vi "Teleop.vi"(10 "Match Info":T1={"Autonomous Elapsed Seconds"=0.0, "TeleOp Elapsed Seconds"=0.0, "Disabled Elapsed Seconds"=0.0, "Visited Autonomous"=FALSE, "Visited TeleOp"=FALSE, "Visited Disabled"=FALSE, "Autonomous Settings"={"Autonomous Style"=enum."Independent", "VI Refnum"=refnum}}, 11 "Call Context":T2) -> ()   [LabVIEW 2019]
doc: "This VI is called for each TeleOp packet received from the DS where the robot is not disabled. It is often used to read from the joysticks and update I/O or to update setpoints for timed control loops. It should complete and return within 20 milliseconds or it may miss DS packets."
uses:
  <vilib>/Rock Robotics/WPI/DriverStation/WPI_DriverStationDerivedRobotMode.ctl
  <vilib>/Rock Robotics/WPI/DriverStation/WPI_DriverStationMatch Info.ctl
  <vilib>/Rock Robotics/WPI/Utilities/WPI_GetSetVariantRefNum.vi
  Robot Global Data.vi
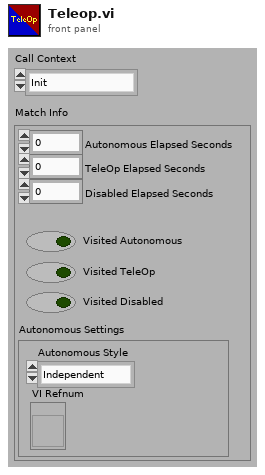
[diagram p1: front panel]
types:
  T1 = typedef "WPI_DriverStationMatch Info.ctl" = cluster{"Autonomous Elapsed Seconds":dbl, "TeleOp Elapsed Seconds":dbl, "Disabled Elapsed Seconds":dbl, "Visited Autonomous":bool, "Visited TeleOp":bool, "Visited Disabled":bool, "Autonomous Settings":cluster{"Autonomous Style":enum16{"Iterative", "Independent"}, "VI Refnum":refnum<vi>}}
  T2 = typedef "WPI_DriverStationDerivedRobotMode.ctl" = enum16{"Init", "Execute", "Stop"}
  T3 = typedef "WPI_JoystickDevRef.ctl" = cluster{"Device":T4}
  T4 = typedef "WPI_JoystickDeviceEnum.ctl" = enum16{"USB 0", "USB 1", "USB 2", "USB 3", "USB 4", "USB 5"}
  T5 = typedef "WPI_RobotDriveDevRef.ctl" = cluster{"DevStatus":errorcluster, "Motors[]":T6[], "Square Inputs":bool, "Max Output":dbl}
  T6 = typedef "WPI_MotorControlDeviceRef.ctl" = cluster{"DeviceStatus":errorcluster, "Type":T7, "PWM":cluster{"PWM Channel":T8, "DeadBand":T9}, "CAN":cluster{"Device Number":u8, "SetOutput VI Ref":variant, "GetOutput VI Ref":variant, "Enable VI Ref":variant, "Disable VI Ref":variant, "Data":variant}, "Invert":bool, "DIO PWM":cluster{"PWM \"Enable\" Channel":T8, "DIOChannel":T10, "PWM Rate":dbl}}
  T7 = typedef "WPI_MotorControlType.ctl" = enum16{"PWM", "CAN", "DIO PWM"}
  T8 = typedef "FPGA_DIOPWMChannel.ctl" = enum8{"PWM 0", "PWM 1", "PWM 2", "PWM 3", "PWM 4", "PWM 5", "PWM 6", "PWM 7", "PWM 8", "PWM 9", "PWM MXP 0", "PWM MXP 1", "PWM MXP 2", "PWM MXP 3", "PWM MXP 4", "PWM MXP 5", "PWM MXP 6", "PWM MXP 7", "PWM MXP 8", "PWM MXP 9", "Invalid"}
  T9 = typedef "WPI_PWMDeadband.ctl" = cluster{"Name":string, "maxPositivePwm":i32, "minPositivePwm":i32, "centerPwm":i32, "maxNegativePwm":i32, "minNegativePwm":i32, "angularRange":u16}
  T10 = typedef "FPGA_DIOChannel.ctl" = enum8{"DIO 0", "DIO 1", "DIO 2", "DIO 3", "DIO 4", "DIO 5", "DIO 6", "DIO 7", "DIO 8", "DIO 9", "DIO MXP 0", "DIO MXP 1", "DIO MXP 2", "DIO MXP 3", "DIO MXP 4", "DIO MXP 5", "DIO MXP 6", "DIO MXP 7", "DIO MXP 8", "DIO MXP 9", "DIO MXP 10", "DIO MXP 11", "DIO MXP 12", "DIO MXP 13", "DIO MXP 14", "DIO MXP 15", "SPI Port CS1", "SPI Port CS2", "SPI Port CS3", "SPI Port MISO", "SPI Port MOSI", "Invalid"}
  T11 = cluster{"JoystickDevRef":T3, "RobotDriveDevRef":T5}
  T12 = typedef "WPI_ServoDeviceRef.ctl" = cluster{"DeviceStatus":errorcluster, "PWM Channel":T8, "DeadBand":T9}
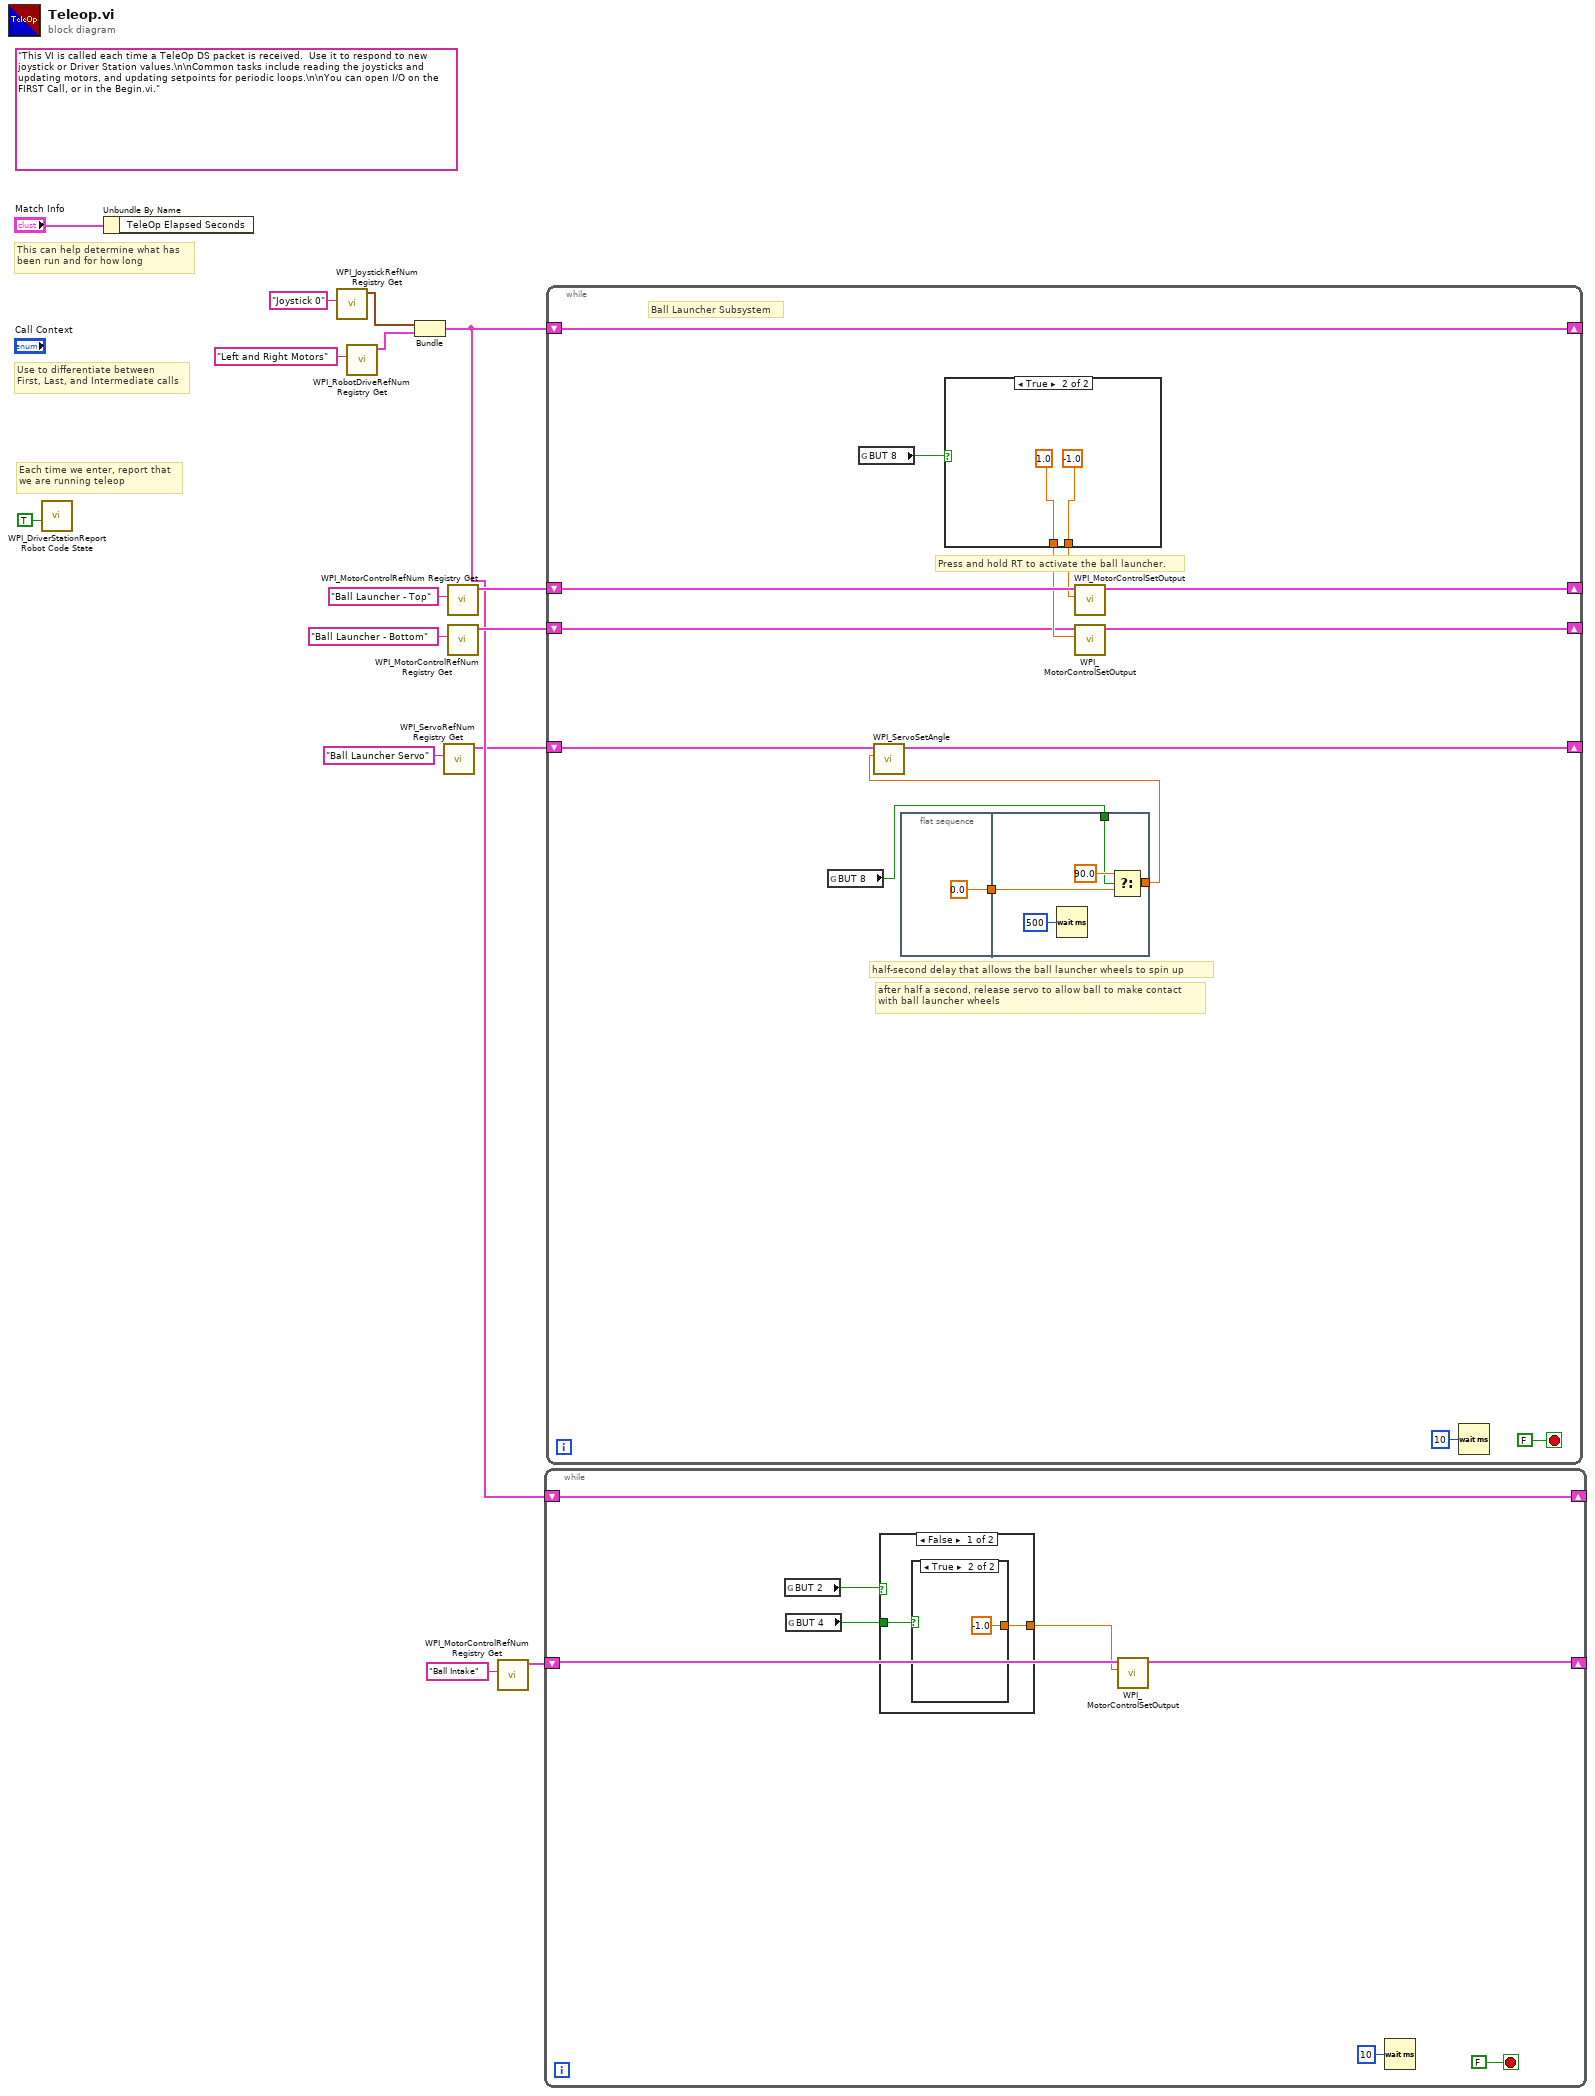
[diagram p0: block diagram]
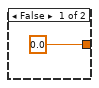
[diagram p2: hidden frame]
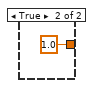
[diagram p3: hidden frame]
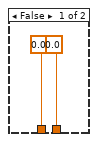
[diagram p4: hidden frame]
diagram:
  (unwired) "This VI is called each time a TeleOp DS packet is received.  Use it to respond to new joystick or Driver Station values.\n\nCommon tasks include reading the joysticks and updating motors, and updating setpoints for periodic loops.\n\nYou can open I/O on the FIRST Call, or in the Begin.vi."
  # "Each time we enter, report that\nwe are running teleop"
  # "Use to differentiate between\nFirst, Last, and Intermediate calls"
  # "This can help determine what has\nbeen run and for how long"
  n1 = call <vilib>:"WPI_DriverStationReport Robot Code State.vi"("TeleOp"=TRUE ("Autonomous")) -> ()  [unwired: 10 in, 1 out]
  n2 = Unbundle By Name("Match Info") -> ()  [unwired: 1 out]
  n3 = call <vilib>:"WPI_JoystickRefNum Registry Get.vi"("refnum name"="Joystick 0") -> ("JoystickDevRef"=w10:T3)  [unwired: 9 in, 1 out]
  n4 = call <vilib>:"WPI_RobotDriveRefNum Registry Get.vi"("refnum name"="Left and Right Motors") -> ("RobotDriveDevRef"=w11:T5)  [unwired: 9 in, 1 out]
  n5 = Bundle("JoystickDevRef"=w10, "RobotDriveDevRef"=w11) -> (w3:T11)  [unwired: 1 in]
  n6 = call <vilib>:"WPI_ServoRefNum Registry Get.vi"("refnum name"="Ball Launcher Servo") -> ("ServoDeviceRef"=w1:T12)  [unwired: 9 in, 1 out]
  n7 = call <vilib>:"WPI_MotorControlRefNum Registry Get.vi"("refnum name"="Ball Launcher - Top") -> ("MotorControlDevRef"=w9:T6)  [unwired: 9 in, 1 out]
  n8 = call <vilib>:"WPI_MotorControlRefNum Registry Get.vi"("refnum name"="Ball Launcher - Bottom") -> ("MotorControlDevRef"=w6:T6)  [unwired: 9 in, 1 out]
  n9 = call <vilib>:"WPI_MotorControlRefNum Registry Get.vi"("refnum name"="Ball Intake") -> ("MotorControlDevRef"=w4:T6)  [unwired: 9 in, 1 out]
  n10 = while {
    shift-right: [w22] -> _
    shift-left: w4 -> [w21]
    shift-right: [w23] -> _
    shift-left: w3 -> [w23]
    stop <- FALSE stop-if-true
    n11 = global read "Robot Global Data.vi" "BUT 2"() -> (w17:bool)
    n12 = global read "Robot Global Data.vi" "BUT 4"() -> (w16:bool)
    n13 = case shown="False" w17 {
      tunnel: [w25 1.0 ("Output")] -> w20
      tunnel: w16 -> [w24 _]
      frame False {
        n14 = case shown="True" w24 {
          tunnel: [0.0 ("Output") -1.0 ("Output")] -> w25
          frame False {
          }
          frame True {
          }
        }
      }
      frame True {
      }
    }
    n15 = call <vilib>:"WPI_MotorControlSetOutput.vi"("Output"=w20, "MotorControlDevRef"=w21) -> ("MotorControlDevRef"=w22:T6)  [unwired: 7 in, 2 out]
    n16 = Wait (ms)(milliseconds to wait=u32 10) -> ()  [unwired: 1 out]
  }
  n17 = while {
    shift-right: [w29] -> _
    shift-left: w3 -> [w29]
    shift-right: [w37] -> _
    shift-left: w9 -> [w42]
    shift-right: [w36] -> _
    shift-left: w6 -> [w38]
    shift-right: [w35] -> _
    shift-left: w1 -> [w33]
    stop <- FALSE stop-if-true
    # "after half a second, release servo to allow ball to make contact\nwith ball launcher wheels"
    # "half-second delay that allows the ball launcher wheels to spin up"
    # "Ball Launcher Subsystem"
    # "Press and hold RT to activate the ball launcher."
    n18 = global read "Robot Global Data.vi" "BUT 8"() -> (w31:bool)
    n19 = global read "Robot Global Data.vi" "BUT 8"() -> (w34:bool)
    n20 = call <vilib>:"WPI_ServoSetAngle.vi"("Angle"=w32, "ServoDeviceRef"=w33) -> ("ServoDeviceRef"=w35:T12)  [unwired: 8 in, 1 out]
    n21 = flat-sequence {
      tunnel: [0.0 ("f")] -> w30
      tunnel: [w48] -> w32
      tunnel: w31 -> [w47]
      tunnel: w30 -> [w45]
      frame #0 {
      }
      frame #1 {
        n22 = Wait (ms)(milliseconds to wait=u32 500) -> ()  [unwired: 1 out]
        n23 = Select(t=90.0, s=w47, f=w45) -> (s? t:f=w48:dbl)
      }
    }
    n24 = case shown="True" w34 {
      tunnel: [0.0 ("Output") -1.0 ("Output")] -> w41
      tunnel: [0.0 ("Output") 1.0 ("Output")] -> w39
      frame False {
      }
      frame True {
      }
    }
    n25 = call <vilib>:"WPI_MotorControlSetOutput.vi"("Output"=w41, "MotorControlDevRef"=w42) -> ("MotorControlDevRef"=w37:T6)  [unwired: 7 in, 2 out]
    n26 = call <vilib>:"WPI_MotorControlSetOutput.vi"("Output"=w39, "MotorControlDevRef"=w38) -> ("MotorControlDevRef"=w36:T6)  [unwired: 7 in, 2 out]
    n27 = Wait (ms)(milliseconds to wait=u32 10) -> ()  [unwired: 1 out]
  }
